vi "Load Project Items.vi"(6 "Clear Existing?":bool, 8 "error in (no error)":errorcluster, 10 "Project Reference":refnum<vi>, 11 "Model in":refnum<class "Model.lvclass">) -> (0 "error out":errorcluster, 3 "Model out":refnum<class "Model.lvclass">)   [LabVIEW 2015, in "Model.lvlib" / "Model.lvclass"]
uses:
  Model.lvclass
  Model Messages/Get VI Infomation Msg/Get VI Infomation Msg.lvclass
  <vilib>/ActorFramework/Actor/Actor.lvclass
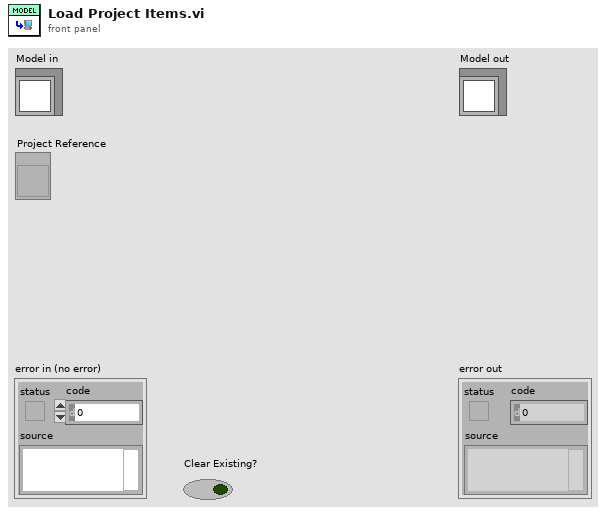
[diagram p1: front panel]
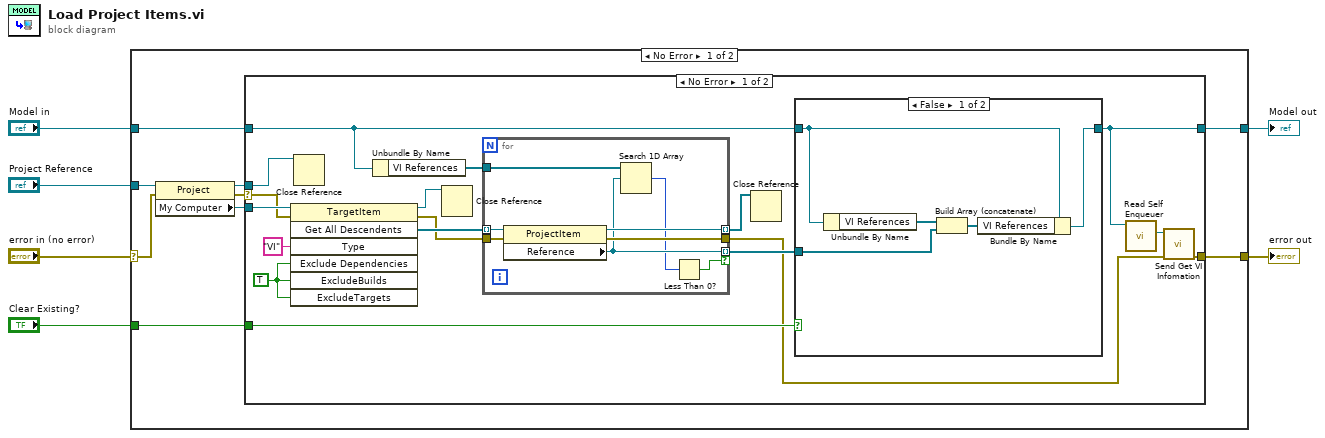
[diagram p0: block diagram]
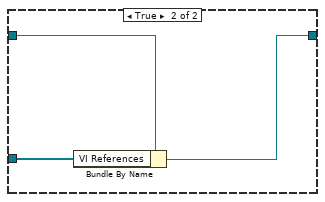
[diagram p2: hidden frame]
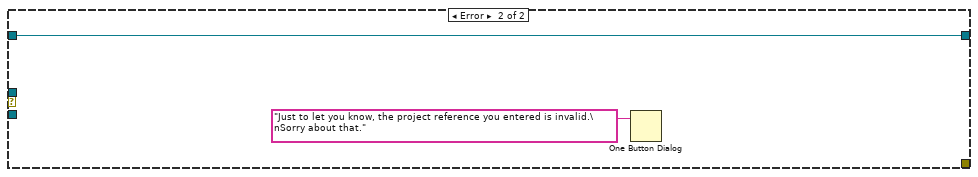
[diagram p3: hidden frame]
diagram:
  n1 = case shown="No Error" "error in (no error)" {
    selector: "error in (no error)" -> [w13 w52]
    tunnel: [w8 w52] -> w5
    tunnel: [w7 w51] -> w3
    tunnel: "Model in" -> [w11 w51]
    tunnel: "Project Reference" -> [w12 _]
    tunnel: "Clear Existing?" -> [w9 _]
    frame No Error {
      n2 = property class="Project"(reference=w12, error in=w13) -> (reference out=w10:refnum<vi>, error out=w14:errorcluster, "My Computer"=w15:refnum<vi>)
      n3 = case shown="No Error" w14 {
        selector: w14 -> [w30 _]
        tunnel: w15 -> [w32 _]
        tunnel: w11 -> [w17 w49]
        tunnel: w10 -> [w26 _]
        tunnel: w9 -> [w23 _]
        tunnel: [w20 _] -> w8
        tunnel: [w19 w49] -> w7
        frame No Error {
          w31 = TRUE ("Exclude dependencies (T)")
          n4 = invoke class="TargetItem" method="Get All Descendents"(reference=w32, error in=w30, "Type"="VI", "Exclude Dependencies"=w31, "ExcludeBuilds"=w31, "ExcludeTargets"=w31) -> (reference out=w25:refnum<vi>, error out=w22:errorcluster, "All Descendents"=w28:refnum<vi>[])  [unwired: 1 in, 4 out]
          n5 = Close Reference(reference=w26) -> ()  [unwired: 1 in, 1 out]
          n6 = Unbundle By Name(w17) -> ("VI References"=w16:refnum<vi>[])
          n7 = Close Reference(reference=w25) -> ()  [unwired: 1 in, 1 out]
          n8 = for {
            tunnel: w28 -> [w40] mode=indexing
            tunnel: [w35] -> w27 mode=indexing if=w33
            tunnel: [w39] -> w24 mode=indexing
            tunnel: w22 -> [w38]
            tunnel: [w37] -> w21
            tunnel: w16 -> [w36]
            n9 = property class="ProjectItem"(reference=w40, error in=w38) -> (reference out=w39:refnum<vi>, error out=w37:errorcluster, "Reference"=w35:refnum<vi>)
            n10 = Search 1D Array(1D array=w36, element=w35) -> (index of element=w34:i32)  [unwired: 1 in]
            n11 = Less Than 0?(x=w34) -> (x < 0?=w33:bool)
          }
          n12 = Close Reference(reference=w24) -> ()  [unwired: 1 in, 1 out]
          n13 = case shown="False" w23 {
            tunnel: w17 -> [w45 w48]
            tunnel: [w44 w47] -> w19
            tunnel: w27 -> [w41 w46]
            frame False {
              n14 = Unbundle By Name(w45) -> ("VI References"=w43:refnum<vi>[])
              n15 = Build Array (concatenate)(w43, w41) -> (w42:refnum<vi>[])
              n16 = Bundle By Name(cluster=w45, "VI References"=w42) -> (w44:refnum<class "Model.lvclass">)
            }
            frame True {
              n17 = Bundle By Name(cluster=w48, "VI References"=w46) -> (w47:refnum<class "Model.lvclass">)
            }
          }
          n18 = call <vilib>:"Read Self Enqueuer.vi"("Actor"=w19) -> ("Self Enqueuer"=w18:refnum<class "Message Enqueuer.lvclass">)  [unwired: 10 in]
          n19 = call "Send Get VI Infomation.vi"("error in (no error)"=w21, "Message Enqueuer"=w18) -> ("error out"=w20:errorcluster)  [unwired: 8 in, 1 out]
        }
        frame Error {
          n20 = One Button Dialog(message="Just to let you know, the project reference you entered is invalid.\nSorry about that.") -> ()  [unwired: 1 in, 1 out]
        }
      }
    }
    frame Error {
    }
  }
  "error out" <- w5
  "Model out" <- w3
